vi "Set Greeter_req.vi"(7 "Complete Call (T)":bool=TRUE, 8 "error in (no error)":errorcluster, 10 "package_templatemessage":T1, 11 "gRPCid":T2) -> (0 "error out":errorcluster)   [LabVIEW 2019, in "Generated_server.lvlib"]
uses:
  Generated_server.lvlib
  <vilib>/gRPC/LabVIEW gRPC Library/Shared/grpcId.ctl
  Greeter_req.ctl
  Greeter_req_req_oneof/Greeter_req_req_oneof.lvclass
  Greeter_req_Flat.ctl
  Greeter_MessageA_Flat.ctl
  Greeter_req_req_oneof/Greeter_req_req_oneof.lvclass/Greeter_req_req_oneof.ctl
  Greeter_MessageA_oneof_a/Greeter_MessageA_oneof_a.lvclass/Greeter_MessageA_oneof_a.ctl
  dcc74a39-081a-4bdd-860b-8ed792803c96.vi
  Greeter_req_req_oneof/GetActiveFieldIndex.vi
  Greeter_req_req_oneof/Getmessage_a.vi
  RichToFlatGreeter_MessageA.vi
  Greeter_req_req_oneof/Getreq_price.vi
  <vilib>/gRPC/LabVIEW gRPC Library/Shared/TranslateGrpcError.vi
  Greeter_MessageA_oneof_a/GetActiveFieldIndex.vi
  Greeter_MessageA_oneof_a/Getdata_a1.vi
  Greeter_MessageA_oneof_a/Getdata_a2.vi
  <vilib>/gRPC/LabVIEW gRPC Library/Server API/Server/Get Server DLL Path.vi
  <vilib>/Utility/error.llb/Error Cluster From Error Code.vi
  <vilib>/Utility/error.llb/Simple Error Handler.vi
  Greeter_MessageA_oneof_a/Greeter_MessageA_oneof_a.lvclass
  <vilib>/gRPC/LabVIEW gRPC Library/grpc-lvsupport-release.lvlib
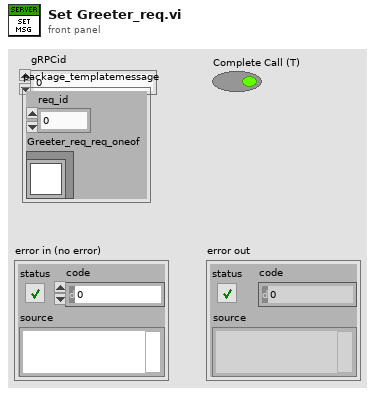
[diagram p1: front panel]
types:
  T1 = typedef "Generated_server.lvlib/Greeter_req.ctl" = cluster{"req_id":i32, "Greeter_req_req_oneof":refnum<class "Greeter_req_req_oneof.lvclass">}
  T2 = typedef "grpc-lvsupport-release.lvlib/grpcId.ctl" = u64
  T3 = typedef "Generated_server.lvlib/Greeter_req_Flat.ctl" = cluster{"req_id":i32, "Greeter_req_req_oneof_selected_index":i32, "message_a":T4, "req_price":dbl}
  T4 = typedef "Generated_server.lvlib/Greeter_MessageA_Flat.ctl" = cluster{"anotherField":string, "Greeter_MessageA_oneof_a_selected_index":i32, "data_a1":string, "data_a2":string}
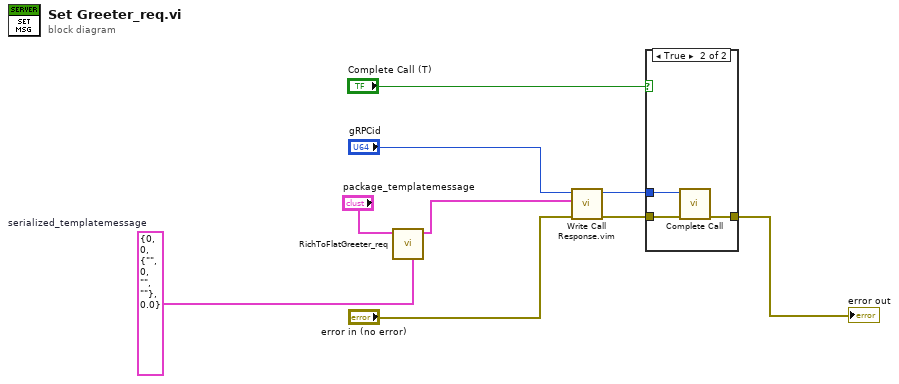
[diagram p0: block diagram]
diagram:
  w2 = T3 {"req_id"=0, "Greeter_req_req_oneof_selected_index"=0, "message_a"={"anotherField"="", "Greeter_MessageA_oneof_a_selected_index"=0, "data_a1"="", "data_a2"=""}, "req_price"=0.0}  # serialized_templatemessage
  n1 = call "RichToFlatGreeter_req.vi"("OutputClusterType"=w2, "InputCluster"="package_templatemessage") -> ("OutputCluster"=w1:T3)  [unwired: 9 in]
  n2 = call "Write Call Response.vim"("error in"="error in (no error)", "Response Data"=w1, "gRPCid in"="gRPCid") -> ("error out"=w6:errorcluster, "gRPCid out"=w7:T2)  [unwired: 7 in]
  n3 = case shown="True" "Complete Call (T)" {
    tunnel: [w10 w13] -> w9
    tunnel: w7 -> [_ w12]
    tunnel: w6 -> [w10 w11]
    frame False {
    }
    frame True {
      n4 = call <vilib>:"Complete Call.vi"("gRPCid"=w12, "error in"=w11) -> ("error out"=w13:errorcluster)  [unwired: 8 in]
    }
  }
  "error out" <- w9
